vi "Duplicate_AO_WF_4Z.vi"(8 "error in (no error)":errorcluster, 11 "AO WF":waveform(dbl)[](graph)=[{"t0"=timestamp(0 s since 1904-01-01), "dt"=0.0001, "Y"=array[9000 elements]}, {"t0"=timestamp(0 s since 1904-01-01), "dt"=0.0001, "Y"=array[9000 elements]}, {"t0"=timestamp(0 s since 1904-01-01), "dt"=0.0001, "Y"=array[9000 elements]}, {"t0"=timestamp(0 s since 1904-01-01), "dt"=0.0001, "Y"=array[9000 elements]}]) -> (0 "error out":errorcluster, 3 "AO WF 2":waveform(dbl)[](graph))   [LabVIEW 2025]
uses:
  <vilib>/Waveform/WDTOps.llb/WDT Append Waveforms DBL.vi
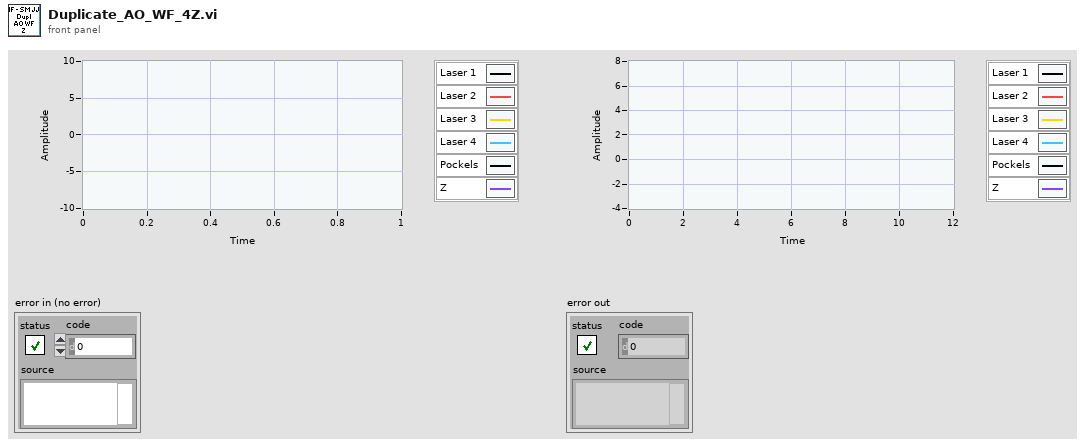
[diagram p1: front panel]
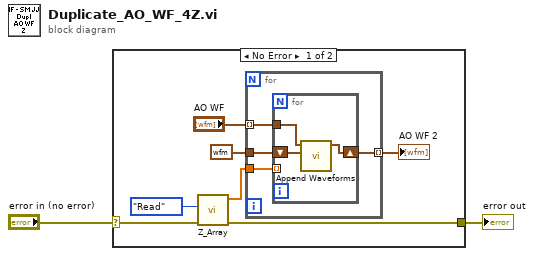
[diagram p0: block diagram]
diagram:
  n1 = case shown="No Error" "error in (no error)" {
    selector: "error in (no error)" -> [w9 w17]
    tunnel: [w7 w17] -> w2
    frame No Error {
      n2 = call "Z_Array.vi"("error in"=w9, "Action"=enum16{"Write", "Read"}."Read") -> ("error out"=w7:errorcluster, "Z_Array"=w3:dbl[])  [unwired: 8 in]
      n3 = for {
        tunnel: "AO WF" -> [w12] mode=indexing
        tunnel: waveform(i32) {"t0"=timestamp(0 s since 1904-01-01), "dt"=1.0, "Y"=[]} ("waveform out") -> [w13]
        tunnel: [w11] -> w5 mode=indexing
        tunnel: w3 -> [w10]
        n4 = for {
          tunnel: w12 -> [w15]
          shift-right: [w14] -> w11
          shift-left: w13 -> [w16]
          tunnel: w10 -> [_] mode=indexing
          n5 = call-poly <vilib>:"Append Waveforms.vi"("waveform B"=w16, "waveform A"=w15) -> ("waveform out"=w14:waveform(dbl))  [unwired: 8 in, 1 out]
        }
      }
      "AO WF 2" <- w5
    }
    frame Error {
    }
  }
  "error out" <- w2
